vi "FPGA Dynamic Ref PoC.vi"() -> ()   [LabVIEW 2024]
uses:
  <vilib>/userDefined/Silver/nirio_resource_slv.ctl
  <vilib>/FPGAPlugInAG/Dynamic/niLvFpga_Close_Dynamic.vi
  <vilib>/rvi/interface/nirviCloseFPGA/nirviCloseFPGA.xnode
  <instrlib>/FlexRIO/API/Host/v1/NI FlexRIO API v1.lvlib
panel:
  in  "Run When Loaded 2":bool
  in  "Run When Loaded":bool
  out "i 2":i32
  out "i":i32
  in  "Close 2":bool
  in  "Init 2":bool
  in  "stop 2":bool
  out "error out 2":errorcluster
  in  "Close":bool
  in  "Init":bool
  in  "stop":bool
  out "error out":errorcluster
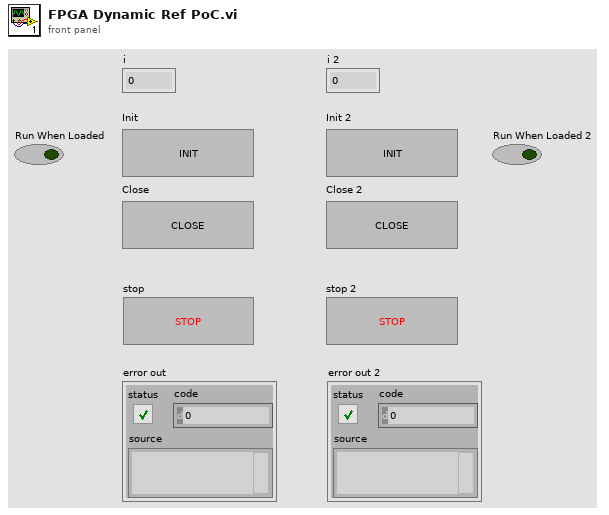
[diagram p1: front panel]
types:
  T1 = typedef "nirio_resource_slv.ctl" = tag
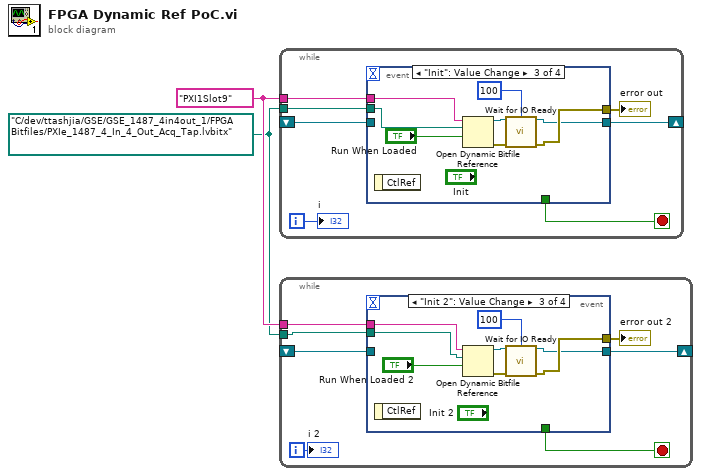
[diagram p0: block diagram]
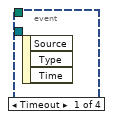
[diagram p2: hidden frame]
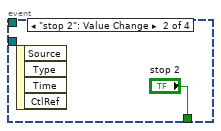
[diagram p3: hidden frame]
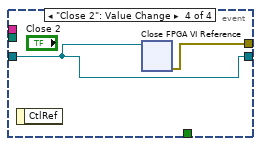
[diagram p4: hidden frame]
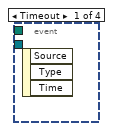
[diagram p5: hidden frame]
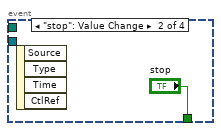
[diagram p6: hidden frame]
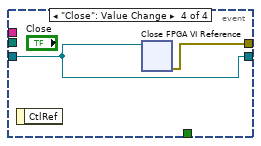
[diagram p7: hidden frame]
diagram:
  w1 = path "C:/dev/ttashjia/GSE/GSE_1487_4in4out_1/FPGA Bitfiles/PXIe_1487_4_In_4_Out_Acq_Tap.lvbitx" ("Bitfile path")
  w2 = T1 "PXI1Slot9" ("RIO Device")
  n1 = while {
    shift-right: [w7] -> _
    shift-left: _ -> [w6]
    tunnel: w2 -> [w5]
    tunnel: w1 -> [w4]
    i -> [w3]
    stop <- w9 stop-if-true
    n2 = event shown="[2] \"Init\": Value Change" {
      selector: _ -> [_ _ _ _]
      dyn-events: _ -> [_ _ _ _]
      timeout: _ -> [_ _ _ _]
      tunnel: [_ "stop" _ _] -> w9
      tunnel: [_ _ w15 w20] -> w8
      tunnel: [_ _ w14 w19] -> w7
      tunnel: w6 -> [_ _ _ w19]
      tunnel: w5 -> [_ _ w13 _]
      tunnel: w4 -> [_ _ w12 _]
      event Timeout {
        n3 = event-data() -> ()  [unwired: 1 in, 3 out]
      }
      event "stop": Value Change {
        n4 = event-data() -> ()  [unwired: 1 in, 4 out]
      }
      event "Init": Value Change {
        n5 = event-data() -> ()  [unwired: 1 in, 1 out]
        n6 = Open Dynamic Bitfile Reference(0:w13, 1:w12, 2:"Run When Loaded") -> (5:w16:refnum<k20>, 8:w17:errorcluster)  [unwired: 2 in]
        n7 = call <instrlib>:"Wait for IO Ready.vi"("fpga interface in"=w16, "timeout"=100, "error in"=w17) -> ("fpga interface out"=w14:refnum<k20>, "error out"=w15:errorcluster)  [unwired: 9 in, 2 out]
      }
      event "Close": Value Change {
        n8 = event-data() -> ()  [unwired: 1 in, 1 out]
        n9 = xnode ("Close FPGA VI Reference")("FPGA VI Reference In"=w19) -> ("error out"=w20:errorcluster)  [unwired: 1 in]
      }
    }
    "error out" <- w8
    "i" <- w3
  }
  n10 = while {
    shift-right: [w25] -> _
    shift-left: _ -> [w24]
    tunnel: w2 -> [w23]
    tunnel: w1 -> [w22]
    i -> [w21]
    stop <- w27 stop-if-true
    n11 = event shown="[2] \"Init 2\": Value Change" {
      selector: _ -> [_ _ _ _]
      dyn-events: _ -> [_ _ _ _]
      timeout: _ -> [_ _ _ _]
      tunnel: [_ "stop 2" _ _] -> w27
      tunnel: [_ _ w33 w38] -> w26
      tunnel: [_ _ w32 w37] -> w25
      tunnel: w24 -> [_ _ _ w37]
      tunnel: w23 -> [_ _ w31 _]
      tunnel: w22 -> [_ _ w30 _]
      event Timeout {
        n12 = event-data() -> ()  [unwired: 1 in, 3 out]
      }
      event "stop 2": Value Change {
        n13 = event-data() -> ()  [unwired: 1 in, 4 out]
      }
      event "Init 2": Value Change {
        n14 = event-data() -> ()  [unwired: 1 in, 1 out]
        n15 = Open Dynamic Bitfile Reference(0:w31, 1:w30, 2:"Run When Loaded 2") -> (5:w34:refnum<k20>, 8:w35:errorcluster)  [unwired: 2 in]
        n16 = call <instrlib>:"Wait for IO Ready.vi"("fpga interface in"=w34, "timeout"=100, "error in"=w35) -> ("fpga interface out"=w32:refnum<k20>, "error out"=w33:errorcluster)  [unwired: 9 in, 2 out]
      }
      event "Close 2": Value Change {
        n17 = event-data() -> ()  [unwired: 1 in, 1 out]
        n18 = xnode ("Close FPGA VI Reference")("FPGA VI Reference In"=w37) -> ("error out"=w38:errorcluster)  [unwired: 1 in]
      }
    }
    "error out 2" <- w26
    "i 2" <- w21
  }
